vi "StopGLOBAL (1).vi"() -> ()   [LabVIEW 2017]
panel:
  out "StopGLOBAL":bool
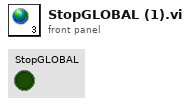
[diagram p1: front panel]
diagram:
